vi "repr_graphical.vi"(9 "Image Descriptor":T1={"Upper-Left Corner Coordinates"={"UTM Zone"=0.0, "Hemisphere"=enum."North", "East"=0.0, "North"=0.0}, "Meters/Pixel"=42.294203} {"Upper-Left Corner Coordinates"."North" format="%#_10f"; "Upper-Left Corner Coordinates"."East" format="%#_8f"}, 10 "Image In":T3, 11 "Mission in":refnum<class "Mission.lvclass">) -> (2 "Image Out":T3, 3 "Mission out":refnum<class "Mission.lvclass">)   [LabVIEW 2011, in "Mission.lvclass"]
doc: "Represents the given mission on an IMAQ image using overlays."
uses:
  Mission.lvclass
  <vilib>/vision/Image Controls.llb/IMAQ Image.ctl
  0-OCU/0 Code/mission input/0-Image Descriptor.ctl
  2 Typedefs/UTM Location.ctl
  Mission.lvclass/Mission.ctl
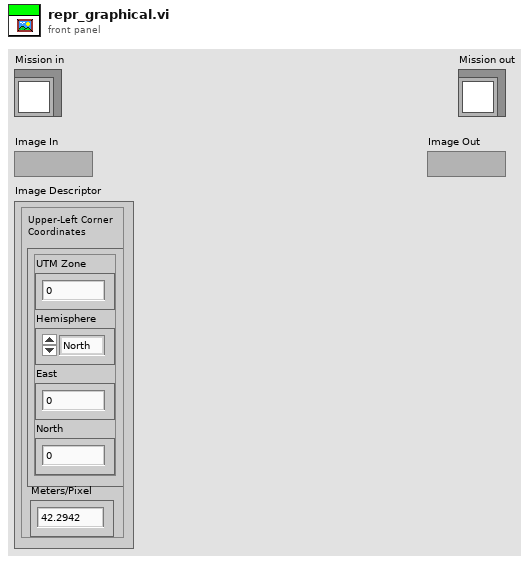
[diagram p1: front panel]
types:
  T1 = typedef "0-Image Descriptor.ctl" = cluster{"Upper-Left Corner Coordinates":T2, "Meters/Pixel":dbl}
  T2 = typedef "UTM Location.ctl" = cluster{"UTM Zone":dbl, "Hemisphere":enum16{"North", "South"}, "East":dbl, "North":dbl}
  T3 = typedef "IMAQ Image.ctl" = refnum<image>
  T4 = enum16{"Round Buoy", "Drive", "Pass Buoys", "Station Keeping"}
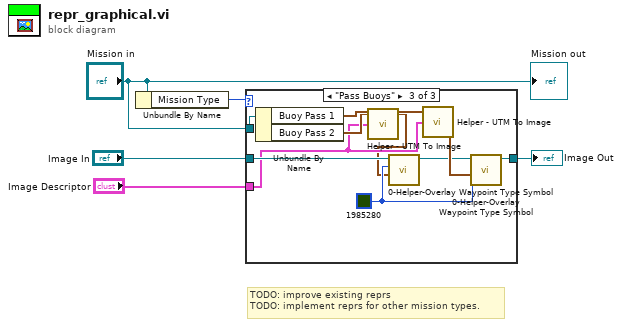
[diagram p0: block diagram]
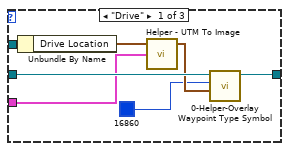
[diagram p2: hidden frame]
diagram:
  # "TODO: improve existing reprs\nTODO: implement reprs for other mission types."
  n1 = Unbundle By Name("Mission in") -> ("Mission Type"=w5:T4)
  n2 = case shown="\"Pass Buoys\"" w5 {
    tunnel: "Image In" -> [w12 w13 w21]
    tunnel: [w11 w13 w22] -> w3
    tunnel: "Image Descriptor" -> [w8 _ w15]
    tunnel: "Mission in" -> [w7 _ w18]
    frame "Drive" {
      n3 = Unbundle By Name(w7) -> ("Drive Location"=w6:T2)
      n4 = call "Helper - UTM To Image.vi"("Image Descriptor"=w8, "UTM Location"=w6) -> ("Pixel Coordinates"=w10:cluster{"X":i32, "Y":i32})  [unwired: 1 in, 2 out]
      n5 = call "0-Helper-Overlay Waypoint Type Symbol.vi"("Overlay Location"=w10, "Icon Color"=u32 16860, "Image in"=w12) -> ("Image out"=w11:T3)  [unwired: 7 in, 1 out]
    }
    frame Default {
    }
    frame "Pass Buoys" {
      w19 = u32 1985280 ("Icon Color")
      n6 = Unbundle By Name(w18) -> ("Buoy Pass 1"=w17:T2, "Buoy Pass 2"=w16:T2)
      n7 = call "Helper - UTM To Image.vi"("Image Descriptor"=w15, "UTM Location"=w16) -> ("Pixel Coordinates"=w14:cluster{"X":i32, "Y":i32})  [unwired: 1 in, 2 out]
      n8 = call "0-Helper-Overlay Waypoint Type Symbol.vi"("Overlay Location"=w14, "Icon Color"=w19, "Image in"=w21) -> ("Image out"=w20:T3)  [unwired: 7 in, 1 out]
      n9 = call "Helper - UTM To Image.vi"("Image Descriptor"=w15, "UTM Location"=w17) -> ("Pixel Coordinates"=w23:cluster{"X":i32, "Y":i32})  [unwired: 1 in, 2 out]
      n10 = call "0-Helper-Overlay Waypoint Type Symbol.vi"("Overlay Location"=w23, "Icon Color"=w19, "Image in"=w20) -> ("Image out"=w22:T3)  [unwired: 7 in, 1 out]
    }
  }
  "Image Out" <- w3
  "Mission out" <- "Mission in"
